vi "pf Set Camera Property S.vi"(8 "error in (no error)":errorcluster, 9 "pValue":string, 10 "pProperty":string, 11 "iPort":i32) -> (0 "error out":errorcluster, 3 "function return":i32)   [LabVIEW 2012, in "Photonfocus_Toolkit.lvlib"]
doc: "PFCONFIG_API int pfSetCameraPropertyS(const char* pProperty, const char* pValue);"
uses:
  <userlib>/Photonfocus Toolkit/Photonfocus_Toolkit.lvlib
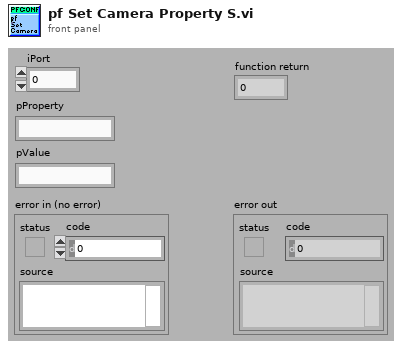
[diagram p1: front panel]
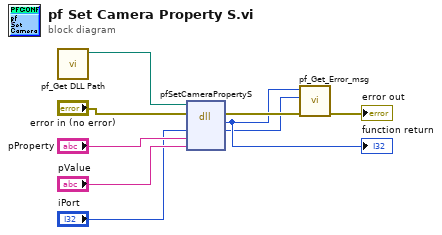
[diagram p0: block diagram]
diagram:
  n1 = call <userlib>:"pf_Get DLL Path.vi"() -> ("DLL path"=w4:path)  [unwired: 1 in, 10 out]
  n2 = dll-call lib="S:/Progetti/Photonfocus/Codice/DEV/PFConfig_lvlib/PFConfig.*" fn="pfSetCameraPropertyS"(path in=w4, error in="error in (no error)", "iPort"="iPort", "pProperty"="pProperty", "pValue"="pValue") -> (error out=w6:errorcluster, "return type"=w2:i32, "iPort"=w1:i32)  [unwired: 3 in, 1 out]
  "function return" <- w2
  n3 = call <userlib>:"pf_Get_Error_msg.vi"("error in (no error)"=w6, "iPort"=w1, "error code"=w2) -> ("error out"=→"error out":errorcluster)  [unwired: 8 out]
